vi "Pre Launch Init.vi"(11 "Sample Line in":refnum<class "Sample Line.lvclass">) -> (0 "error out":errorcluster, 3 "Sample Line out":refnum<class "Sample Line.lvclass">)   [LabVIEW 2015, in "cRIO-Carbondioxide.lvlib" / "CO2-Actor.lvlib" / "Sample Line.lvclass"]
doc: "(<B>Filename</B>: Actor Framework.lvlib:Actor.lvclass:Pre Launch Init.vi)\n\nDefines behavior that occurs after the Launch Actor method is invoked but before the actor's Actor Core method begins running.\n\nThe Pre Launch Init method is guaranteed to finish before the Launch Actor method returns to its caller and before the actor itself receives any messages. Any references that the Pre Launch Init method obtains are guaranteed to have the same lifetime as the actor itself. Any errors that the Pre Launch Init method returns will abort the launch.\n\nBy default, this method does nothing. A descendant class may override it to define behavior."
uses:
  Sample Line.lvclass
  Controls/Sample Line State Enumerator.ctl
  <vilib>/ActorFramework/Message Enqueuer/Message Priority.ctl
  Sample Line.lvclass/Sample Line.ctl
  <vilib>/ActorFramework/Actor/Actor.lvclass/Actor.ctl
  <vilib>/ActorFramework/Message Enqueuer/Message Enqueuer.lvclass/Message Enqueuer.ctl
  <vilib>/ActorFramework/Actor/Read Self Enqueuer.vi
  <vilib>/ActorFramework/Message Enqueuer/Enqueue.vi
  <vilib>/ActorFramework/Message Enqueuer/Init from Existing Queue.vi
  <vilib>/ActorFramework/Message Priority Queue/Priority Enqueue.vi
  CO2 Actor/CO2 Actor.lvclass
  Sample Line Messages/Launch Valves Msg/Launch Valves Msg.lvclass
  <vilib>/ActorFramework/Message Enqueuer/Message Enqueuer.lvclass
  <vilib>/ActorFramework/Actor/Actor.lvclass
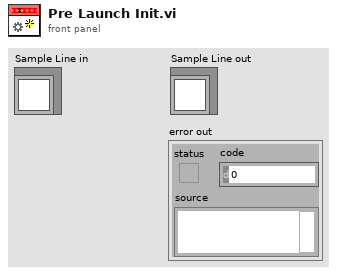
[diagram p1: front panel]
types:
  T1 = typedef "Actor Framework.lvlib/Message Enqueuer.lvclass/Message Priority.ctl" = enum16{"Low", "Normal", "High"}
  T2 = typedef "Sample Line State Enumerator.ctl" = enum16{"All lines closed", "Sample line 1.", "Sample line 2.", "Sample line 3.", "Sample line 4.", "Sample line 5.", "Out of range"}
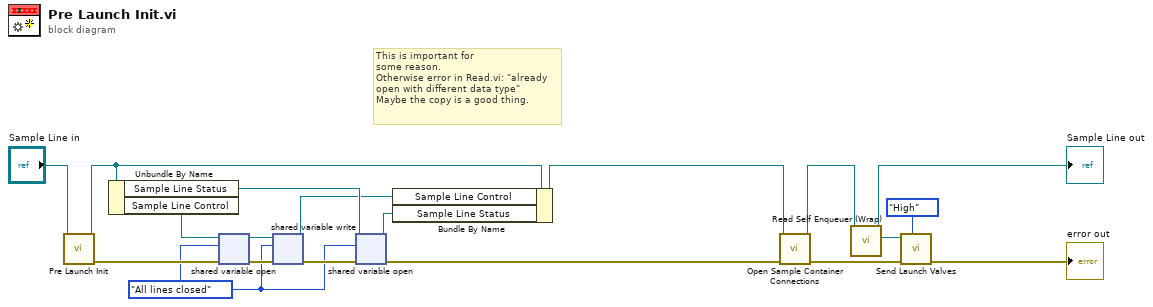
[diagram p0: block diagram]
diagram:
  w11 = Sample_Line_State_Enumerator."All lines closed" ("Enum")
  # "This is important for\nsome reason.\nOtherwise error in Read.vi: \"already\nopen with different data type\"\nMaybe the copy is a good thing."
  n1 = call-parent "Pre Launch Init.vi"("CO2 Actor in"="Sample Line in") -> ("error out"=w15:errorcluster, "CO2 Actor out"=w17:refnum<class "Sample Line.lvclass">)  [unwired: 9 in]
  n2 = Unbundle By Name(w17) -> ("Sample Line Status"=w14:refnum<k21>, "Sample Line Control"=w16:refnum<k21>)
  n3 = shared-variable-open(w16, w15, w11) -> (w10:refnum<k21>, w13:errorcluster)  [unwired: 1 in]
  n4 = shared-variable-write(w10, w13, w11) -> (w9:refnum<k21>, w12:errorcluster)
  n5 = shared-variable-open(w14, w12, w11) -> (w3:refnum<k21>, w2:errorcluster)  [unwired: 1 in]
  n6 = Bundle By Name(cluster=w17, "Sample Line Control"=w9, "Sample Line Status"=w3) -> (w1:refnum<class "Sample Line.lvclass">)
  n7 = call "Open Sample Container Connections.vi"("error in (no error)"=w2, "Sample Line in"=w1) -> ("error out"=w7:errorcluster, "Sample Line out"=w8:refnum<class "Sample Line.lvclass">)  [unwired: 8 in]
  n8 = call "Read Self Enqueuer (Wrap).vi"("CO2 Actor in"=w8) -> ("Actor Framework:Message Enqueuer"=w18:refnum<class "Message Enqueuer.lvclass">, "CO2 Actor out"=→"Sample Line out":refnum<class "Sample Line.lvclass">)  [unwired: 9 in]
  n9 = call "Send Launch Valves.vi"("Message Priority (Normal)"=Message_Priority."High", "error in (no error)"=w7, "Message Enqueuer"=w18) -> ("error out"=→"error out":errorcluster)  [unwired: 7 in, 1 out]
